vi "Create Flex Channel.vi"(6 "Item Path":path, 7 "app":refnum<vi>, 11 "Element Type":variant) -> (0 "error IO":errorcluster, 3 "Channel Control Path":path)   [LabVIEW 2022 SP3, in "FlexBlocks Support.lvlib"]
uses:
  FlexBlocks Support.lvlib
  <resource>/ChannelSupport/_ChannelScriptingSupport/_ChannelScriptingSupport.lvlib
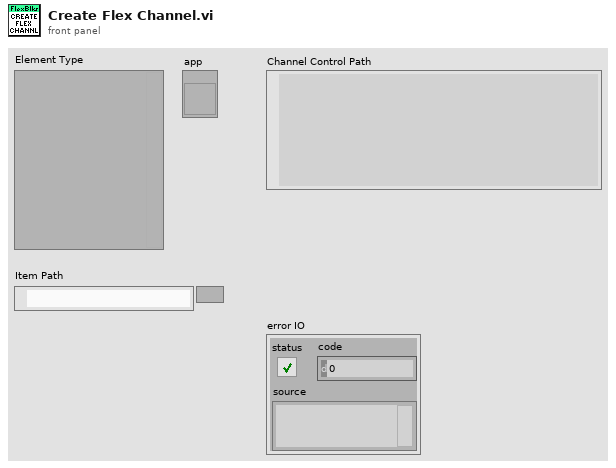
[diagram p1: front panel]
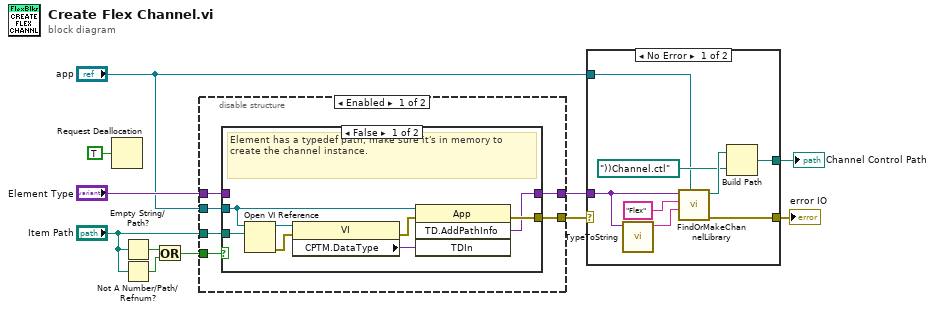
[diagram p0: block diagram]
diagram:
  n1 = Request Deallocation(TRUE ("flag")) -> ()
  n2 = Empty String/Path?(string/path="Item Path") -> (empty?=w11:bool)
  n3 = Not A Number/Path/Refnum?(number/path/refnum="Item Path") -> (NaN/Path/Refnum?=w10:bool)
  n4 = Or(x=w11, y=w10) -> (x .or. y?=w5:bool)
  n5 = disable-structure shown="Enabled" {
    disable-tunnel: "Item Path" -> [w17 _]
    disable-tunnel: "Element Type" -> [w16 w27]
    disable-tunnel: [w15 _] -> w7
    disable-tunnel: [w14 w27] -> w6
    disable-tunnel: w5 -> [w13 _]
    disable-tunnel: "app" -> [w12 _]
    frame Enabled {
      n6 = case shown="False" w13 {
        tunnel: w17 -> [w24 _]
        tunnel: w16 -> [_ w26]
        tunnel: [w18 w26] -> w14
        tunnel: w12 -> [w21 _]
        tunnel: [w20 _] -> w15
        frame False {
          # "Element has a typedef path, make sure it's in memory to create the channel instance."
          n7 = Open VI Reference(application reference (local)=w21, vi path=w24) -> (vi reference=w23:refnum<vi>, error out=w22:errorcluster)  [unwired: 4 in]
          n8 = property class="VI"(reference=w23, error in=w22) -> (error out=w25:errorcluster, "CPTM.DataType"=w19:variant)  [unwired: 1 out]
          n9 = invoke class="App" method="TD.AddPathInfo"(reference=w21, error in=w25, "TDIn"=w19) -> (error out=w20:errorcluster, "TD.AddPathInfo"=w18:variant)  [unwired: 1 in, 2 out]
        }
        frame True {
          # "Element is not a typedef, can create channel directly from it."
        }
      }
    }
    frame Disabled {
    }
  }
  n10 = case shown="No Error" w7 {
    selector: w7 -> [_ w36]
    tunnel: "app" -> [w29 _]
    tunnel: w6 -> [w28 _]
    tunnel: [w30 _] -> w3
    tunnel: [w35 w36] -> w2
    frame No Error {
      n11 = call <resource>:"TypeToString.vi"("type"=w28) -> ("string"=w33:string)  [unwired: 10 in]
      n12 = call <resource>:"FindOrMakeChannelLibrary.vi"("app"=w29, "typestring"=w33, "class"="Flex", "elt type"=w28) -> ("error out"=w35:errorcluster, "channel folder"=w32:path)  [unwired: 6 in]
      n13 = Build Path(base path=w32, name or relative path=path "))Channel.ctl") -> (appended path=w30:path)
    }
    frame Error {
    }
  }
  "Channel Control Path" <- w3
  "error IO" <- w2
